vi "Add Event.vi"(6 "Source Has Handler (F)":bool, 8 "error in (no error)":errorcluster, 9 "Source Event Fire Handler":refnum<class "Abstract Source Event Handler.lvclass">, 10 "Event":refnum<class "Event.lvclass">, 11 "Event Source in":refnum<class "Event Source.lvclass">) -> (0 "error out":errorcluster, 3 "Event Source out":refnum<class "Event Source.lvclass">)   [LabVIEW 2016, in "Event Source.lvlib" / "Event Source.lvclass"]
doc: "This methods adds an event to the list of the events handled by the source. If the source wants to handle events form the sink a \"Source Event Fire Handler\" can wired and the booleant input \"Source has Handler\" set to True"
uses:
  Event Source.lvclass
  Event/Event.lvclass
  Event Source Messages/Abstract Source Event Handler/Abstract Source Event Handler.lvclass
  Event Source.lvclass/Event Source.ctl
  <vilib>/Utility/error.llb/Error Cluster From Error Code.vi
  <vilib>/ErrorRing/Error Ring.xnode
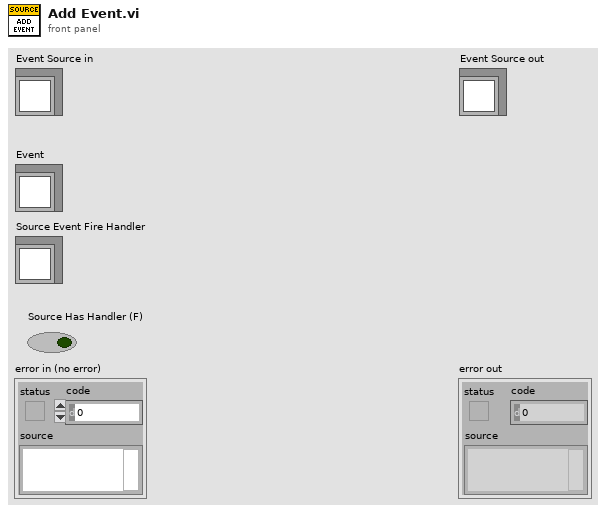
[diagram p1: front panel]
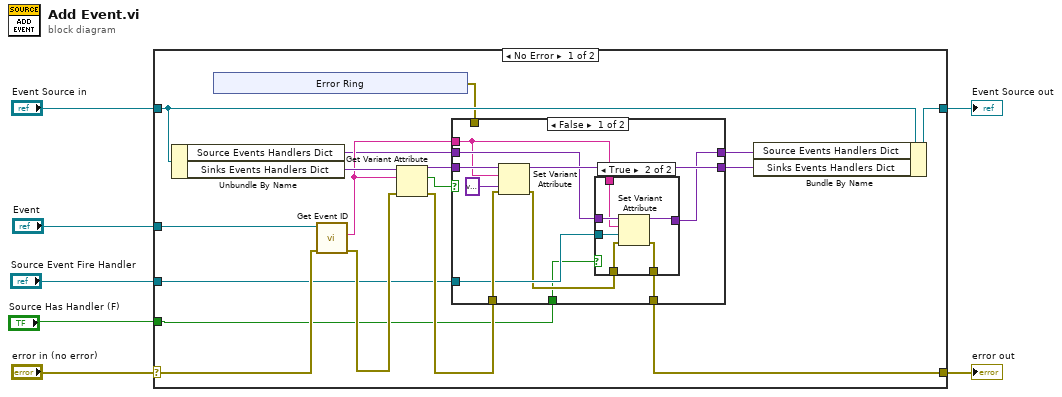
[diagram p0: block diagram]
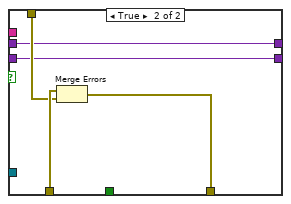
[diagram p3: hidden frame]
diagram:
  n1 = case shown="No Error" "error in (no error)" {
    selector: "error in (no error)" -> [w22 w54]
    tunnel: [w10 w54] -> w6
    tunnel: [w14 w53] -> w4
    tunnel: "Event Source in" -> [w24 w53]
    tunnel: "Event" -> [w23 _]
    tunnel: "Source Event Fire Handler" -> [w11 _]
    tunnel: "Source Has Handler (F)" -> [w9 _]
    frame No Error {
      n2 = Unbundle By Name(w24) -> ("Source Events Handlers Dict"=w12:variant, "Sinks Events Handlers Dict"=w21:variant)
      n3 = xnode "Error Ring"() -> ("error out"=w15:errorcluster)
      n4 = call-dynamic "Get Event ID.vi"("error in (no error)"=w22, "Event in"=w23) -> ("error out"=w20:errorcluster, "Event ID"=w17:string)  [unwired: 7 in, 1 out]
      n5 = Get Variant Attribute(Variant=w21, name=w17, error in=w20) -> (duplicate Variant=w18:variant, found=w19:bool, error out=w16:errorcluster)  [unwired: 1 in, 1 out]
      n6 = case shown="False" w19 {
        tunnel: w18 -> [w39 w50]
        tunnel: w17 -> [w34 _]
        tunnel: w16 -> [w38 w52]
        tunnel: w15 -> [_ w51]
        tunnel: [w36 w50] -> w13
        tunnel: w12 -> [w35 w48]
        tunnel: w11 -> [w33 _]
        tunnel: [w31 w49] -> w10
        tunnel: w9 -> [w30 _]
        tunnel: [w29 w48] -> w8
        frame False {
          n7 = Set Variant Attribute(Variant=w39, name=w34, value=variant ("Events Dict"), error in=w38) -> (Variant out=w36:variant, error out=w32:errorcluster)  [unwired: 1 out]
          n8 = case shown="True" w30 {
            tunnel: w35 -> [w40 w47]
            tunnel: w34 -> [_ w46]
            tunnel: w33 -> [_ w45]
            tunnel: w32 -> [w41 w44]
            tunnel: [w41 w43] -> w31
            tunnel: [w40 w42] -> w29
            frame False {
            }
            frame True {
              n9 = Set Variant Attribute(Variant=w47, name=w46, value=w45, error in=w44) -> (Variant out=w42:variant, error out=w43:errorcluster)  [unwired: 1 out]
            }
          }
        }
        frame True {
          n10 = Merge Errors(w52, w51) -> (w49:errorcluster)
        }
      }
      n11 = Bundle By Name(cluster=w24, "Source Events Handlers Dict"=w8, "Sinks Events Handlers Dict"=w13) -> (w14:refnum<class "Event Source.lvclass">)
    }
    frame Error {
    }
  }
  "error out" <- w6
  "Event Source out" <- w4
